vi "Create_Object.vi"(8 "error in (no error)":errorcluster, 9 "Terminal Map in":map{string, T1}(c390), 10 "owner refnum":variant, 11 "Case Selector in":refnum<class "Case Structure.lvclass">) -> (0 "error out":errorcluster, 1 "Terminal Map Out":map{string, T1}(c390), 3 "Case Selector out":refnum<class "Case Structure.lvclass">)   [LabVIEW 2025, in "Case Structure.lvclass"]
uses:
  Case Structure.lvclass
  Controls/Terminal.ctl
  Node.lvclass/Node.ctl
  MultiDiagramStructure.lvclass
  Node.lvclass
panel:
  out "size(s)":i32
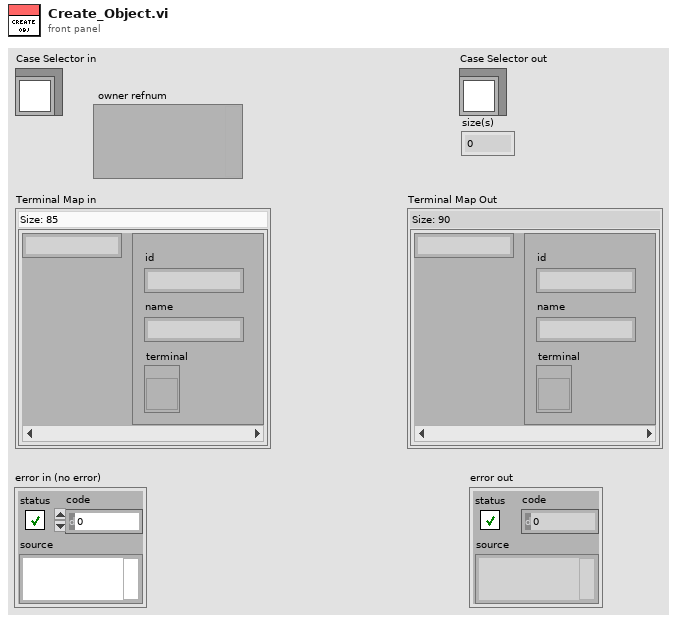
[diagram p1: front panel]
types:
  T1 = typedef "Terminal.ctl" = cluster{"id":string, "name":string, "terminal":refnum<vi>}
  T2 = typedef "Subdiagram.ctl" = cluster{"diagram":refnum<vi>, "selector":string, "uuid":string}
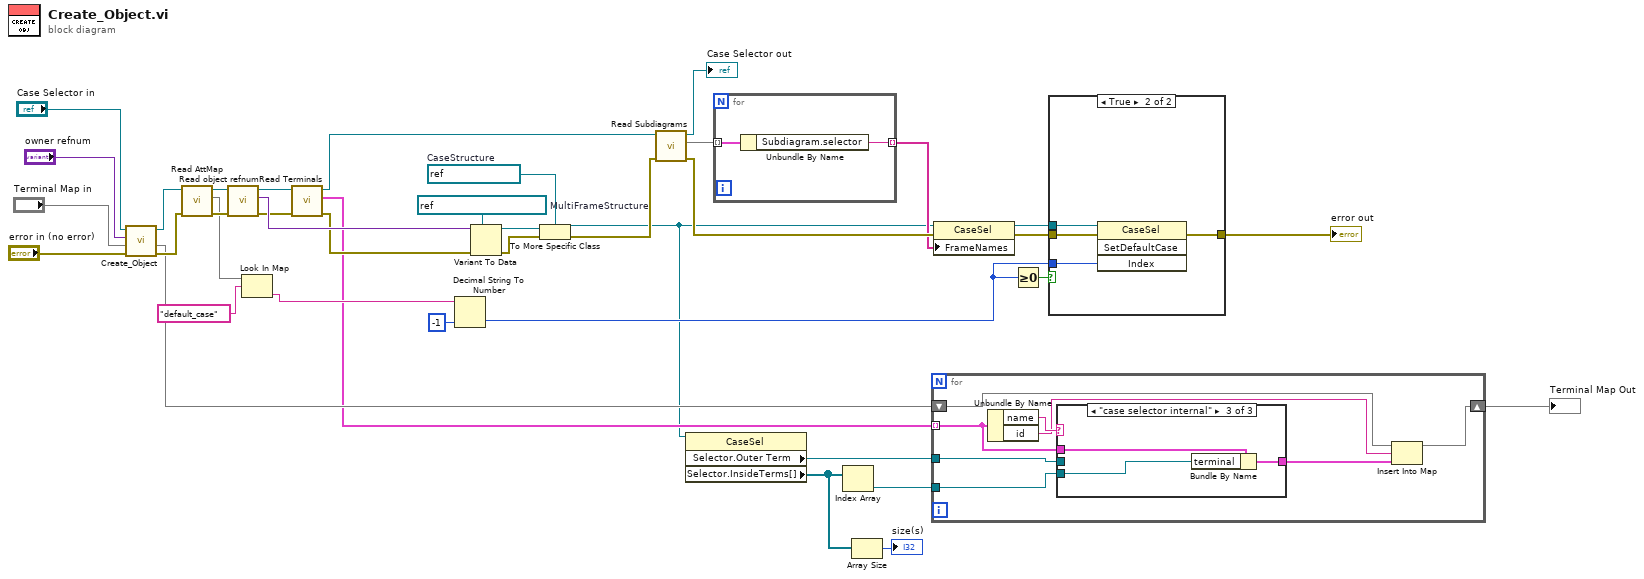
[diagram p0: block diagram]
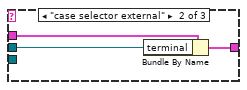
[diagram p3: hidden frame]
diagram:
  w26 = refnum<vi> refnum  # CaseStructure
  w28 = refnum<vi> refnum  # MultiFrameStructure
  n1 = call-parent "Create_Object.vi"("error in (no error)"="error in (no error)", "Terminal Map in"="Terminal Map in", "owner refnum"="owner refnum", "MultiDiagramStructure in"="Case Selector in") -> ("error out"=w35:errorcluster, "Terminal Map Out"=w11:map{string, T1}, "MultiDiagramStructure out"=w34:refnum<class "Case Structure.lvclass">)  [unwired: 5 in]
  n2 = call "Read AttMap.vi"("error in (no error)"=w35, "Node in"=w34) -> ("error out"=w33:errorcluster, "AttMap"=w30:map{string, string}, "Node out"=w32:refnum<class "Case Structure.lvclass">)  [unwired: 7 in]
  n3 = call-dynamic "Read object refnum.vi"("error in (no error)"=w33, "Node in"=w32) -> ("error out"=w8:errorcluster, "object refnum"=w29:variant, "Node out"=w10:refnum<class "Case Structure.lvclass">)  [unwired: 7 in]
  n4 = Look In Map(map=w30, key="default_case") -> (value=w20:string)  [unwired: 1 in, 1 out]
  n5 = call "Read Terminals.vi"("error in (no error)"=w8, "Node in"=w10) -> ("error out"=w7:errorcluster, "Terminals"=w6:T1[], "Node out"=w9:refnum<class "Case Structure.lvclass">)  [unwired: 7 in]
  n6 = Decimal String To Number(string=w20, default (0L)=-1 ("default (0 I32)")) -> (number=w15:i32)  [unwired: 1 in, 1 out]
  n7 = Variant To Data(error in=w7, type=w28, Variant=w29) -> (data=w27:refnum<vi>, error out=w25:errorcluster)
  n8 = To More Specific Class(target class=w26, reference=w27, error in=w25) -> (specific class reference=w5:refnum<vi>, error out=w23:errorcluster)
  n9 = call-dynamic "Read Subdiagrams.vi"("error in (no error)"=w23, "MultiDiagramStructure in"=w9) -> ("error out"=w22:errorcluster, "Subdiagrams"=w24:map{u64, T2}, "MultiDiagramStructure out"=→"Case Selector out":refnum<class "Case Structure.lvclass">)  [unwired: 7 in]
  n10 = property class="CaseSel"(reference=w5) -> ("Selector.Outer Term"=w14:refnum<vi>, "Selector.InsideTerms[]"=w2:refnum<vi>[])  [unwired: 1 in, 2 out]
  n11 = for {
    tunnel: w24 -> [w41] mode=indexing
    tunnel: [w40] -> w21 mode=indexing
    n12 = Unbundle By Name(w41) -> ("Subdiagram.selector"=w40:string)
  }
  n13 = Index Array(array=w2) -> (element=w13:refnum<vi>)  [unwired: 1 in]
  n14 = Array Size(array=w2) -> (size(s)=→"size(s)":i32)
  n15 = for {
    tunnel: w6 -> [w42] mode=indexing
    tunnel: w14 -> [w46]
    shift-right: [w48] -> w12
    shift-left: w11 -> [w49]
    tunnel: w13 -> [w44]
    n16 = Unbundle By Name(w42) -> ("name"=w47:string, "id"=w45:string)
    n17 = case shown="\"case selector internal\"" w47 {
      tunnel: w46 -> [_ w51 _]
      tunnel: w44 -> [_ _ w54]
      tunnel: [w50 w53 w55] -> w43
      tunnel: w42 -> [w50 w52 w56]
      frame "False", Default {
      }
      frame "case selector external" {
        n18 = Bundle By Name(cluster=w52, "terminal"=w51) -> (w53:T1)
      }
      frame "case selector internal" {
        n19 = Bundle By Name(cluster=w56, "terminal"=w54) -> (w55:T1)
      }
    }
    n20 = Insert Into Map(map in=w49, key=w45, value=w43) -> (map out=w48:map{string, T1})  [unwired: 2 out]
  }
  "Terminal Map Out" <- w12
  n21 = property class="CaseSel"(reference=w5, error in=w22, "FrameNames"=w21) -> (reference out=w16:refnum<vi>, error out=w17:errorcluster)
  n22 = Greater Or Equal To 0?(x=w15) -> (x >= 0?=w18:bool)
  n23 = case shown="True" w18 {
    tunnel: w17 -> [w57 w61]
    tunnel: w16 -> [_ w60]
    tunnel: w15 -> [_ w59]
    tunnel: [w57 w58] -> w4
    frame False {
    }
    frame True {
      n24 = invoke class="CaseSel" method="SetDefaultCase"(reference=w60, error in=w61, "Index"=w59) -> (error out=w58:errorcluster)  [unwired: 1 in, 3 out]
    }
  }
  "error out" <- w4
